vi "Get Menus.vi"(8 "error in (no error)":errorcluster, 10 "Message type":string) -> (0 "error out":errorcluster, 1 "Left Menu":T1, 2 "Right Menu":T1)   [LabVIEW 2019]
uses:
  controls/Left Right Menu.ctl
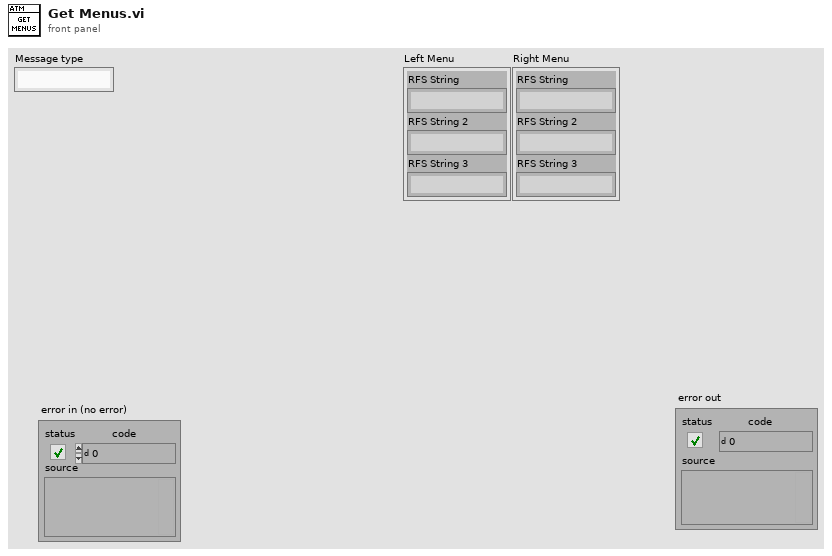
[diagram p1: front panel]
types:
  T1 = cluster{"RFS String":string, "RFS String 2":string, "RFS String 3":string}
  T2 = typedef "Left Right Menu.ctl" = cluster{"Message type":string, "Left Menu":cluster{"RFS String":string, "RFS String 2":string, "RFS String 3":string}, "Right Menu":cluster{"RFS String":string, "RFS String 2":string, "RFS String 3":string}}[]
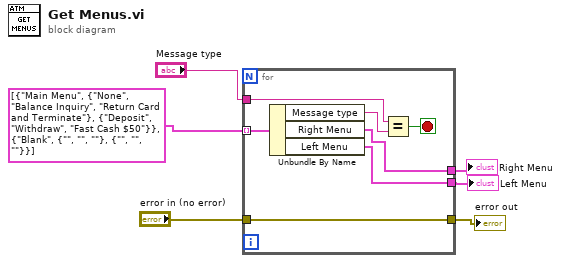
[diagram p0: block diagram]
diagram:
  n1 = for {
    tunnel: T2 [{"Message type"="Main Menu", "Left Menu"={"RFS String"="None", "RFS String 2"="Balance Inquiry", "RFS String 3"="Return Card and Terminate"}, "Right Menu"={"RFS String"="Deposit", "RFS String 2"="Withdraw", "RFS String 3"="Fast Cash $50"}}, {"Message type"="Blank", "Left Menu"={"RFS String"="", "RFS String 2"="", "RFS String 3"=""}, "Right Menu"={"RFS String"="", "RFS String 2"="", "RFS String 3"=""}}] ("Menu Strings") -> [w13] mode=indexing
    tunnel: "Message type" -> [w12]
    tunnel: "error in (no error)" -> [w9]
    tunnel: [w9] -> w4
    tunnel: [w8] -> w1
    tunnel: [w7] -> w2
    stop <- w10 stop-if-true
    n2 = Unbundle By Name(w13) -> ("Message type"=w11:string, "Right Menu"=w7:T1, "Left Menu"=w8:T1)
    n3 = Equal?(x=w12, y=w11) -> (x = y?=w10:bool)
  }
  "error out" <- w4
  "Left Menu" <- w1
  "Right Menu" <- w2
